vi "Fault List 2 Array.vi"(9 "Fault List":T2[](array[typedef]), 10 "LBCB Number":T1, 11 "DofType":T5) -> (2 "Faults":bool[](array[boolean]))   [LabVIEW 2009]
uses:
  Data Access Objects/Limits/DofTypes.ctl
  Fault Id.ctl
  Fault Type.ctl
  Data Access Objects/Metadata/LBCB Number.ctl
  Space Type.ctl
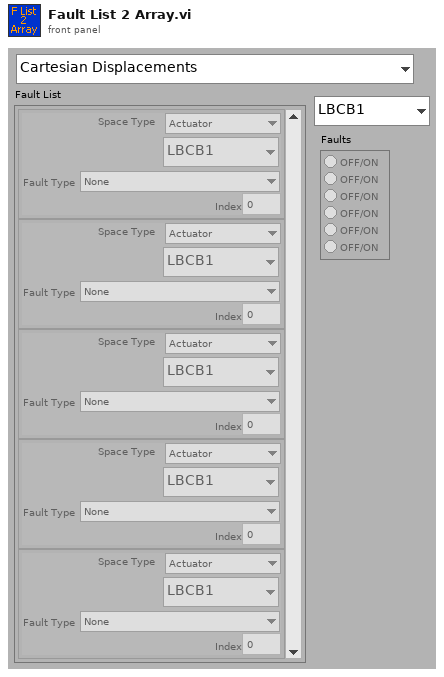
[diagram p1: front panel]
types:
  T1 = typedef "LBCB Number.ctl" = enum16{"LBCB1", "LBCB2"}
  T2 = typedef "Fault Id.ctl" = cluster{"Fault Type":T3, "LBCB Number":T1, "Index":u32, "Space Type":T4}
  T3 = typedef "Fault Type.ctl" = enum16{"None", "Command", "Displacement", "Force", "Increment"}
  T4 = typedef "Space Type.ctl" = enum16{"Actuator", "Cartesian"}
  T5 = typedef "DofTypes.ctl" = enum16{"Cartesian Displacements", "Cartesian Forces & Moments", "Actuator Displacements", "Actuator Forces", "Cartesian Increments", "Actuator Increments"}
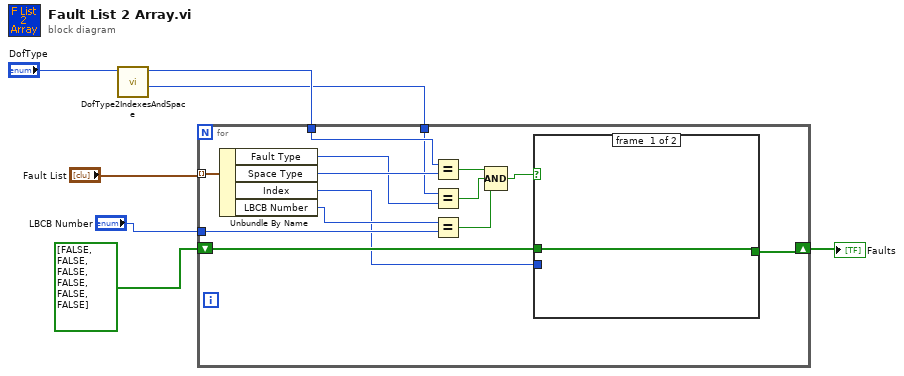
[diagram p0: block diagram]
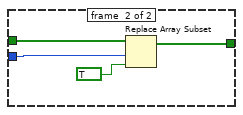
[diagram p2: hidden frame]
diagram:
  n1 = call "DofType2IndexesAndSpace.vi"("DofType"="DofType") -> ("Fault Type"=w1:T3, "Space Type"=w6:T4)  [unwired: 9 in]
  n2 = for {
    tunnel: "Fault List" -> [w21] mode=indexing
    tunnel: w6 -> [w19]
    shift-right: [w15] -> w4
    shift-left: bool[] [FALSE, FALSE, FALSE, FALSE, FALSE, FALSE] ("Faults") -> [w16]
    tunnel: "LBCB Number" -> [w13]
    tunnel: w1 -> [w9]
    n3 = Unbundle By Name(w21) -> ("Fault Type"=w10:T3, "Space Type"=w20:T4, "Index"=w11:u32, "LBCB Number"=w14:T1)
    n4 = Equal?(x=w19, y=w20) -> (x = y?=w18:bool)
    n5 = Equal?(x=w9, y=w10) -> (x = y?=w8:bool)
    n6 = Equal?(x=w14, y=w13) -> (x = y?=w12:bool)
    n7 = Compound Arithmetic op=AND(w18, w8, w12) -> (w17:bool)
    n8 = case shown="True" w17 {
      tunnel: w16 -> [w22 w26]
      tunnel: w11 -> [_ w25]
      tunnel: [w22 w23] -> w15
      frame #0 {
      }
      frame #1 {
        n9 = Replace Array Subset(array=w26, new element=TRUE ("new element/subarray"), index=w25) -> (w23:bool[])
      }
    }
  }
  "Faults" <- w4
